vi "SCD - Check if Exposure Time is Permitted with Desired FPS.vi"(6 "Andor":T1={"Handle"=0, "Pixel Encoding"="", "AOI Width"=0, "AOI Height"=0, "AOI Stride"=0, "Row Readout Time"=0.0, "Frame Readout Time"=0.0, "Interframe Time"=0.0, "Semaphore"=refnum, "SerialNumber"="", "Camera Model"="", "Controller ID"="", "Firmware Version"="", "Shutter"="Global", "BDiv"=1, "Time at Synch"=timestamp(3029526000.379448 s since 1904-01-01), "Idx"=0, "PreAmp"="", "Binning"=enum."1x1", "PixelReadoutRate"="", "Exposure (s)"=0.05, "Image Bytes"=0, "Image Pixels"=0, "SpuriousNoiseFilter"=FALSE, "Overlap"=FALSE, "CycleMode"=""} {"Exposure (s)" format="%^.3g"; "Time at Synch" format="%<%H:%M:%S>T"; "Interframe Time" format="%#_3g"; "Frame Readout Time" format="%_3g"; "Row Readout Time" format="%_3g"}, 7 "Set Exp or Check Fps (Set Exp)":enum16{"Set Exp", "Check FPS"}(ring), 8 "error in (no error)":errorcluster, 11 "Exposure [s]":dbl) -> (0 "error out":errorcluster, 3 "FPS":dbl=1.0)   [LabVIEW 2014]
doc: "Use this template to build a VI to use as a subVI."
uses:
  Camera/Andor Neo Info.ctl
  Controls/beaning.ctl
panel:
  out "FPS out":dbl=25.0 format="%.2f"
  out "Is Camera Exposure Acceptable":bool
  out "Maximum Exposure [ms]":dbl
  in  "FPS in":dbl=25.0 format="%0.2p"
  # "disabled"
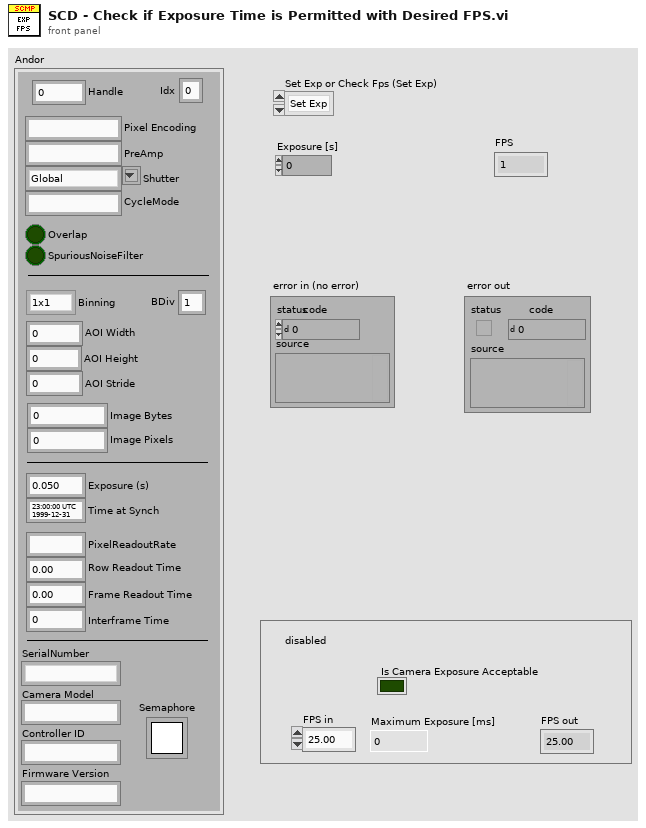
[diagram p1: front panel]
types:
  T1 = typedef "Andor Neo Info.ctl" = cluster{"Handle":i32, "Pixel Encoding":string, "AOI Width":i32, "AOI Height":i32, "AOI Stride":i32, "Row Readout Time":dbl, "Frame Readout Time":dbl, "Interframe Time":dbl, "Semaphore":T2, "SerialNumber":string, "Camera Model":string, "Controller ID":string, "Firmware Version":string, "Shutter":string, "BDiv":u8, "Time at Synch":timestamp, "Idx":i32, "PreAmp":string, "Binning":T3, "PixelReadoutRate":string, "Exposure (s)":dbl, "Image Bytes":i64, "Image Pixels":i64, "SpuriousNoiseFilter":bool, "Overlap":bool, "CycleMode":string}
  T2 = typedef "Semaphore RefNum" = refnum<k1>
  T3 = typedef "beaning.ctl" = enum16{"1x1", "2x2", "3x3", "4x4", "8x8"}
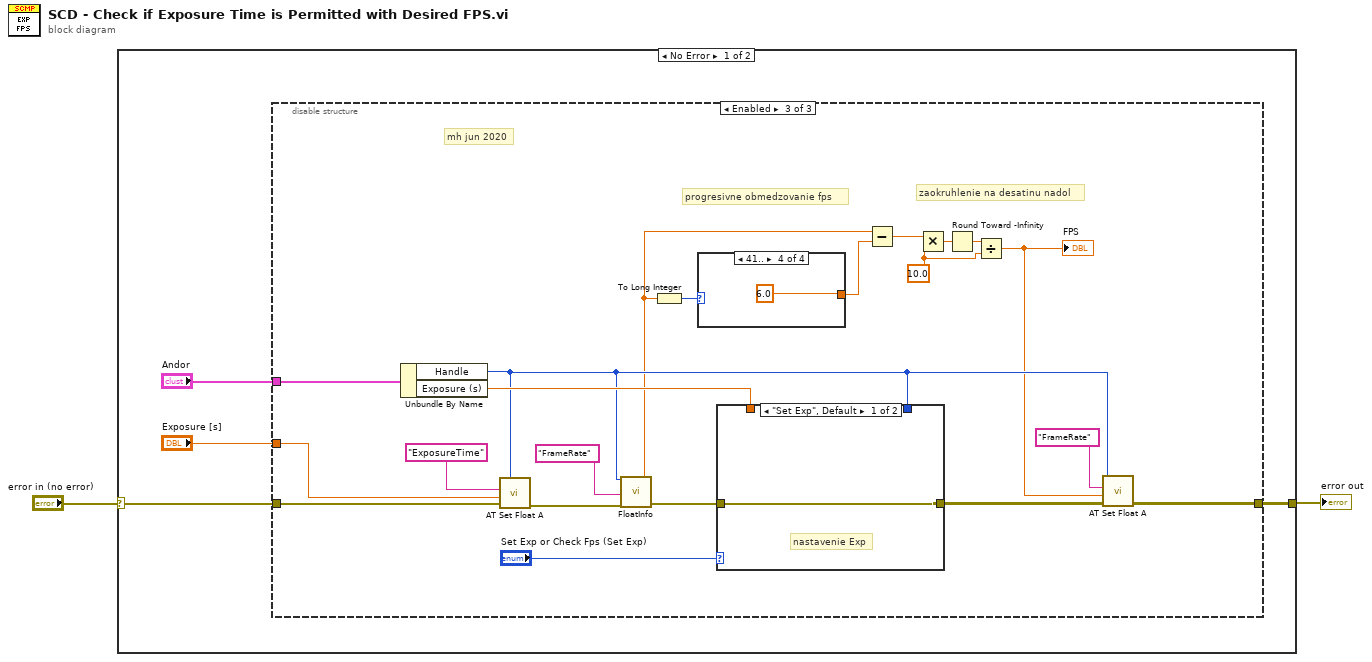
[diagram p0: block diagram]
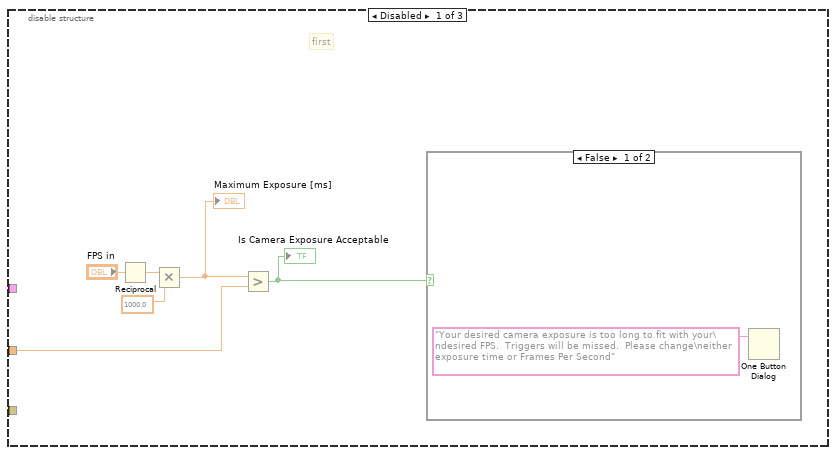
[diagram p2: hidden frame]
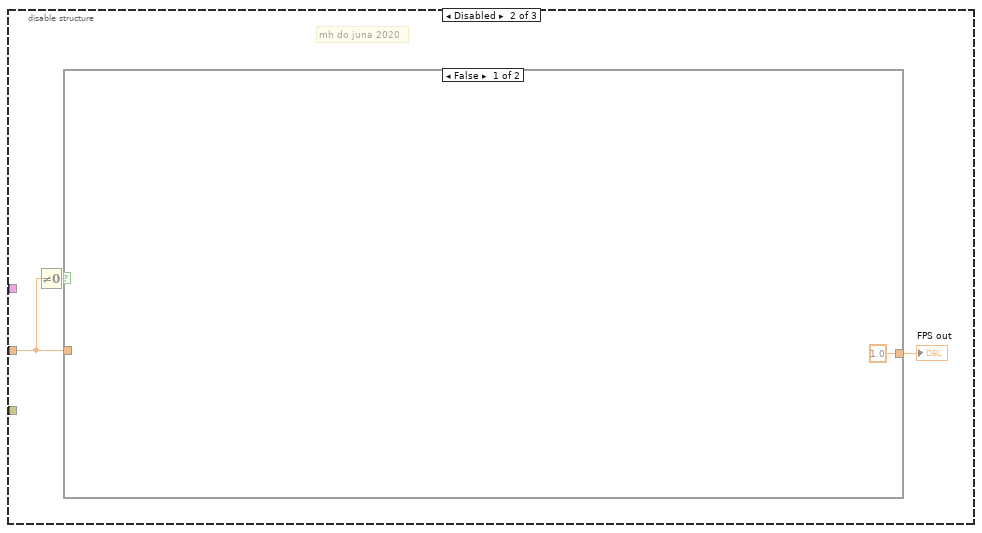
[diagram p4: hidden frame]
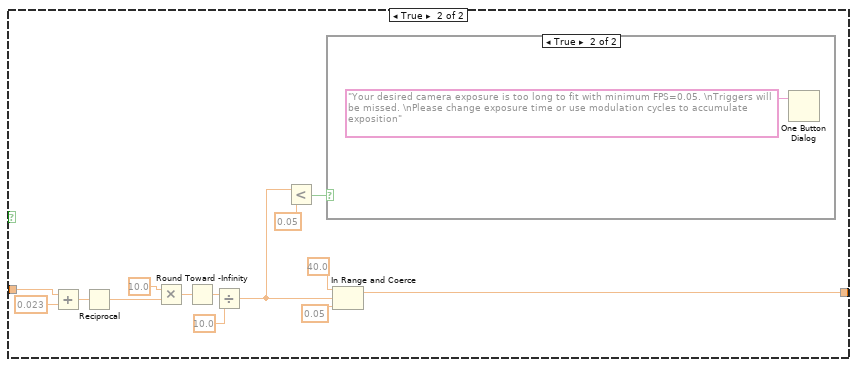
[diagram p5: hidden frame]
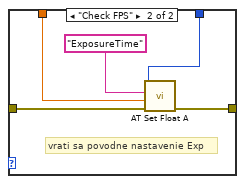
[diagram p7: hidden frame]
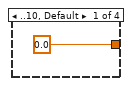
[diagram p8: hidden frame]
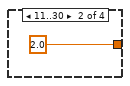
[diagram p9: hidden frame]
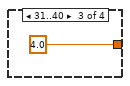
[diagram p10: hidden frame]
diagram:
  n1 = case shown="No Error" "error in (no error)" {
    selector: "error in (no error)" -> [w5 w64]
    tunnel: [w4 w64] -> w1
    frame No Error {
      n2 = disable-structure shown="Enabled" {
        disable-tunnel: "Exposure [s]" -> [w7 w15 w48]
        disable-tunnel: w5 -> [_ _ w52]
        disable-tunnel: [_ _ w38] -> w4
        disable-tunnel: "Andor" -> [_ _ w47]
        frame Disabled {
          # "first"
          n3 = Reciprocal(x="FPS in") -> (1/x=w11:dbl)
          n4 = Multiply(x=w11, y=1000.0) -> (x*y=w9:dbl)
          "Maximum Exposure [ms]" <- w9
          n5 = Greater?(x=w9, y=w7) -> (0:w8:bool)
          "Is Camera Exposure Acceptable" <- w8
          n6 = case shown="False" w8 {
            frame False {
              n7 = One Button Dialog(message="Your desired camera exposure is too long to fit with your\ndesired FPS.  Triggers will be missed.  Please change\neither exposure time or Frames Per Second") -> ()  [unwired: 1 in, 1 out]
            }
            frame True {
              # "Camera Exposure will fit between trigger pulses set by FPS"
            }
          }
        }
        frame Disabled {
          # "mh do juna 2020"
          n8 = Not Equal To 0?(x=w15) -> (x != 0?=w16:bool)
          n9 = case shown="False" w16 {
            tunnel: w15 -> [_ w31]
            tunnel: [1.0 ("upper limit") w18] -> w14
            frame False {
            }
            frame True {
              n10 = Add(x=w31, y=0.023) -> (x+y=w28:dbl)
              n11 = Reciprocal(x=w28) -> (1/x=w29:dbl)
              n12 = Multiply(x=10.0, y=w29) -> (x*y=w27:dbl)
              n13 = Round Toward -Infinity(1:w27) -> (0:w24:dbl)
              n14 = Divide(x=w24, y=10.0) -> (x/y=w19:dbl)
              n15 = Less?(x=w19, y=0.05) -> (x < y?=w20:bool)
              n16 = case shown="True" w20 {
                frame False {
                }
                frame True {
                  n17 = One Button Dialog(message="Your desired camera exposure is too long to fit with minimum FPS=0.05. \nTriggers will be missed. \nPlease change exposure time or use modulation cycles to accumulate exposition") -> ()  [unwired: 1 in, 1 out]
                }
              }
              n18 = In Range and Coerce(upper limit=40.0, x=w19, lower limit=0.05) -> (coerced(x)=w18:dbl)  [unwired: 1 out]
            }
          }
          "FPS out" <- w14
        }
        frame Enabled {
          w41 = 10.0 ("y")
          # "zaokruhlenie na desatinu nadol"
          # "progresivne obmedzovanie fps"
          # "mh jun 2020"
          n19 = Unbundle By Name(w47) -> ("Handle"=w37:i32, "Exposure (s)"=w46:dbl)
          n20 = call <userlib>:"AT Set Float A.vi"("error in (no error)"=w52, "Value"=w48, "Feature"="ExposureTime", "Hndl"=w37) -> ("error out"=w51:errorcluster)  [unwired: 6 in, 1 out]
          n21 = call <userlib>:"FloatInfo.vi"("Handle"=w37, "Feature"="FrameRate", "error in (no error)"=w51) -> ("error out"=w49:errorcluster, "Max"=w34:dbl)  [unwired: 10 in, 5 out]
          n22 = To Long Integer(number=w34) -> (32bit integer=w40:i32)
          n23 = case shown="41.." w40 {
            tunnel: [0.0 2.0 4.0 6.0] -> w45
            frame ..10, Default {
            }
            frame 11..30 {
            }
            frame 31..40 {
            }
            frame 41.. {
            }
          }
          n24 = case shown="\"Set Exp\", Default" "Set Exp or Check Fps (Set Exp)" {
            tunnel: w49 -> [w54 w59]
            tunnel: w46 -> [_ w57]
            tunnel: [w54 w56] -> w39
            tunnel: w37 -> [_ w55]
            frame "Set Exp", Default {
              # "nastavenie Exp"
            }
            frame "Check FPS" {
              # "vrati sa povodne nastavenie Exp"
              n25 = call <userlib>:"AT Set Float A.vi"("error in (no error)"=w59, "Value"=w57, "Feature"="ExposureTime", "Hndl"=w55) -> ("error out"=w56:errorcluster)  [unwired: 6 in, 1 out]
            }
          }
          n26 = Subtract(x=w34, y=w45) -> (x-y=w44:dbl)
          n27 = Multiply(x=w44, y=w41) -> (x*y=w43:dbl)
          n28 = Round Toward -Infinity(1:w43) -> (0:w42:dbl)
          n29 = Divide(x=w42, y=w41) -> (x/y=w35:dbl)
          "FPS" <- w35
          n30 = call <userlib>:"AT Set Float A.vi"("error in (no error)"=w39, "Value"=w35, "Feature"="FrameRate", "Hndl"=w37) -> ("error out"=w38:errorcluster)  [unwired: 6 in, 1 out]
        }
      }
    }
    frame Error {
    }
  }
  "error out" <- w1
